vi "templates import template.vi"(8 "error in (no error)":errorcluster, 9 "Content (\"\")":string, 10 "user":string, 11 "Connection Refnum":T3) -> (0 "error out":errorcluster, 1 "template parameters":T1, 2 "New Template Record":T2, 3 "Connection Refnum":T3)   [LabVIEW 2011]
uses:
  Summitek EXT/ODBC/SQL Controls/Connection Refnum.ctl
  server/database/Templates/Template Record.ctl
  ITK EXT/utils/keyedarr.llb/Keyed Array.ctl
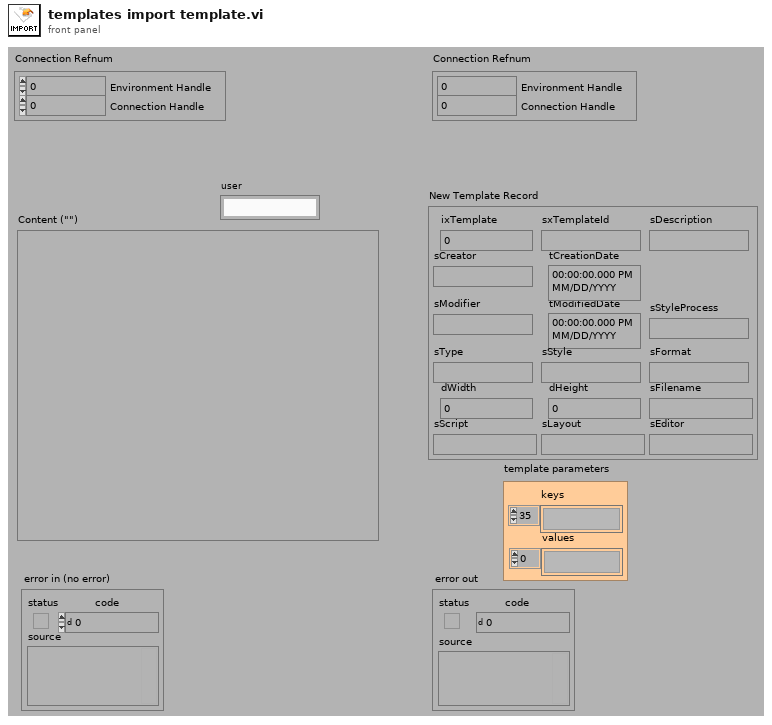
[diagram p1: front panel]
types:
  T1 = typedef "Keyed Array.ctl" = cluster{"keys":string[], "values":string[]}
  T2 = typedef "Template Record.ctl" = cluster{"ixTemplate":i32, "sxTemplateId":string, "sDescription":string, "sCreator":string, "tCreationDate":timestamp, "sModifier":string, "tModifiedDate":timestamp, "sType":string, "sStyle":string, "sFormat":string, "dWidth":dbl, "dHeight":dbl, "sFilename":string, "sScript":string, "sLayout":string, "sEditor":string, "sStyleProcess":string}
  T3 = typedef "Connection Refnum.ctl" = cluster{"Environment Handle":i32, "Connection Handle":i32}
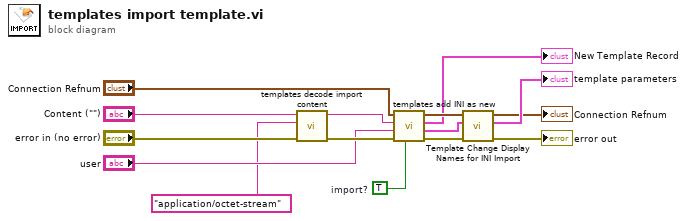
[diagram p0: block diagram]
diagram:
  w10 = TRUE  # import?
  n1 = call "templates decode import content.vi"("error in (no error)"="error in (no error)", "Valid Content-Type: (\"text/xml\")"="application/octet-stream" ("Valid Content-Type: (\"text/xml\")"), "Multi-Part Content (\"\")"="Content (\"\")") -> ("error out"=w6:errorcluster, "Content"=w8:string)  [unwired: 7 out]
  n2 = call "templates add INI as new.vi"("import?"=w10, "error in"=w6, "user"="user", "INI File Content"=w8, "Connection Refnum"="Connection Refnum") -> ("error out"=w11:errorcluster, "Parameters"=w13:T1, "updated Template Record"=→"New Template Record":T2, "Connection Refnum 2"=w14:T3)  [unwired: 3 out]
  n3 = call "Template Change Display Names for INI Import.vi"("error in (no error)"=w11, "Parameters"=w13, "Connection Refnum"=w14) -> ("error out"=→"error out":errorcluster, "Parameters 2"=→"template parameters":T1, "Connection Refnum 2"=→"Connection Refnum":T3)  [unwired: 6 out]
